vi "Close User Config.vi"(8 "error in (no error)":errorcluster) -> (0 "error out":errorcluster)   [LabVIEW 2014]
uses:
  <vilib>/Utility/config.llb/NI_LVConfig.lvlib
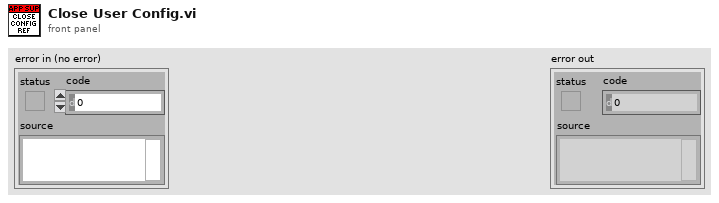
[diagram p1: front panel]
types:
  T1 = typedef "NI_LVConfig.lvlib/Config Data RefNum.ctl" = refnum<k1>
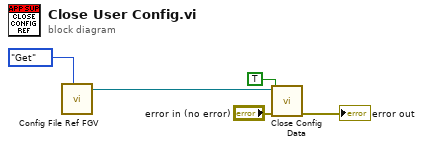
[diagram p0: block diagram]
diagram:
  n1 = call "Config File Ref FGV.vi"("Method"=enum16{"Get", "Set"}."Get") -> ("config refnum out"=w4:T1)  [unwired: 10 in]
  n2 = call <vilib>:"Close Config Data.vi"("error in (no error)"="error in (no error)", "write file if changed (T)"=TRUE, "refnum"=w4) -> ("error out"=→"error out":errorcluster)  [unwired: 7 in, 1 out]
